vi "Init(Config) Log Text File Sink.vi"(7 "Text File Sink Configuration":T1, 8 "error in (no error)":errorcluster, 9 "iName":string, 10 "iType":string) -> (0 "error out":errorcluster, 3 "Text File Sink out":refnum<class "Text File Sink.lvclass">)   [LabVIEW 2016, in "Stream Log.lvlib" / "Text File Sink.lvclass"]
doc: "--\nCopyright © 2017 Composed SystemsI All rights reserved.\n\nAuthor: Jon McBee <jon.mcbee@composed.io>\n\nThis library is provided \"AS IS\" ,WITHOUT WARRANTIES OR\nCONDITIONS OF ANY KIND, either express or implied.\n\nComposed Systems -- composed.io\n\nStream 0.0.1.1\nJon McBee - Composed Systems\nCopyright (c) 2017, Composed Systems"
uses:
  <userlib>/Composed Systems/Stream/Log/Text File Sink/Text File Sink.lvclass
  C:/Program Files (x86)/National Instruments/LabVIEW 2016/user.lib/Composed Systems/Stream/Actor/Actor Class/Ancestral Actor.lvclass
  <userlib>/Composed Systems/Stream/Log/Text File Sink/Configuration.ctl
  <userlib>/Composed Systems/Stream/Actor/Actor Class/Ancestral Actor.lvclass/Ancestral Actor.ctl
  <userlib>/Composed Systems/Stream/Log/Text File Sink/Text File Sink.lvclass/Text File Sink.ctl
  <userlib>/Composed Systems/Stream/Actor/Actor Class/Ancestral Actor.lvclass
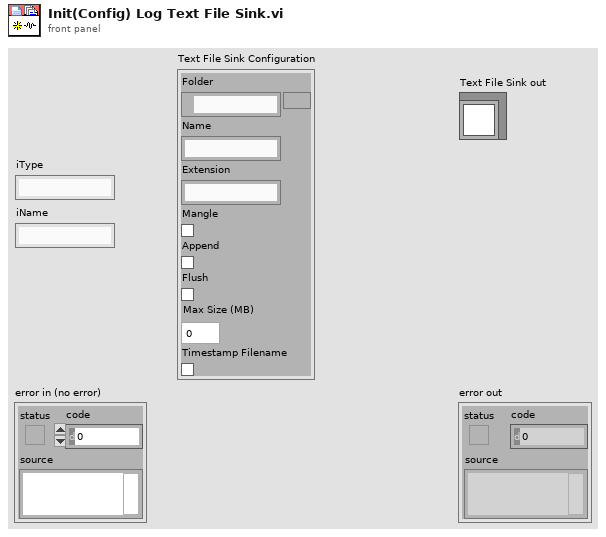
[diagram p1: front panel]
types:
  T1 = typedef "Stream Log.lvlib/Text File Sink.lvclass/Configuration.ctl" = cluster{"Folder":path, "Name":string, "Extension":string, "Mangle":bool, "Append":bool, "Flush":bool, "Max Size (MB)":i64, "Timestamp Filename":bool}
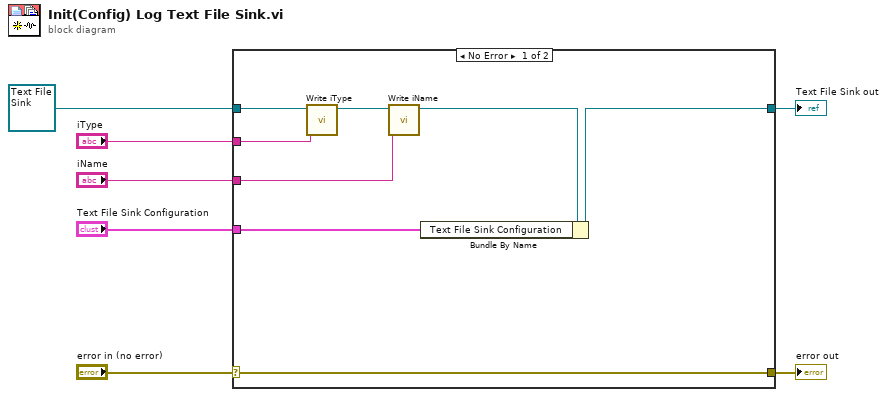
[diagram p0: block diagram]
diagram:
  n1 = case shown="No Error" "error in (no error)" {
    selector: "error in (no error)" -> [w15 w17]
    tunnel: [w15 w17] -> w6
    tunnel: [w13 w16] -> w4
    tunnel: refnum<class "Text File Sink.lvclass"> refnum ("Text File Sink in") -> [w12 w16]
    tunnel: "Text File Sink Configuration" -> [w14 _]
    tunnel: "iType" -> [w11 _]
    tunnel: "iName" -> [w8 _]
    frame No Error {
      n2 = call <userlib>:"Write iType.vi"("iType"=w11, "Ancestral Actor in"=w12) -> ("Ancestral Actor out"=w10:refnum<class "Text File Sink.lvclass">)  [unwired: 8 in, 1 out]
      n3 = call <userlib>:"Write iName.vi"("iName"=w8, "Ancestral Actor in"=w10) -> ("Ancestral Actor out"=w9:refnum<class "Text File Sink.lvclass">)  [unwired: 8 in, 1 out]
      n4 = Bundle By Name(cluster=w9, "Text File Sink Configuration"=w14) -> (w13:refnum<class "Text File Sink.lvclass">)
    }
    frame Error {
    }
  }
  "error out" <- w6
  "Text File Sink out" <- w4
